vi "保存下载配置.vi"(10 "输入数组":string[][](array[string])) -> ()   [LabVIEW 2016]
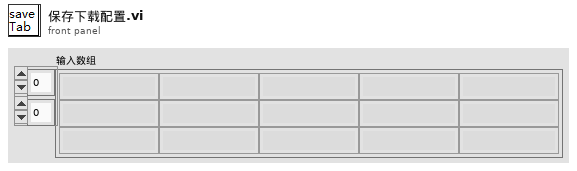
[diagram p1: front panel]
types:
  T1 = enum16{"open", "replace", "create", "open or create", "replace or create", "replace or create with confirmation"}
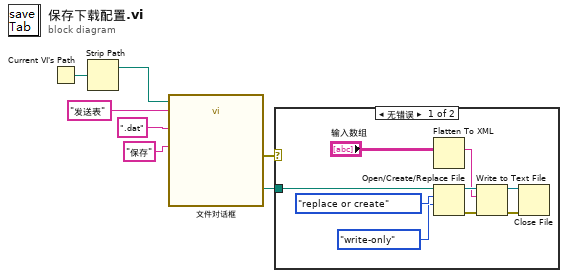
[diagram p0: block diagram]
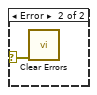
[diagram p2: hidden frame]
diagram:
  n1 = Current VI's Path() -> (path=w7:path)
  n2 = Strip Path(path=w7) -> (stripped path=w1:path)  [unwired: 1 out]
  n3 = call "文件对话框"("start path"=w1, "button label"="保存", "default name"="发送表" ("名称或相对路径"), "pattern (all files)"=".dat") -> ("selected path"=w3:path, "error out"=w2:errorcluster)  [unwired: 8 in, 2 out]
  n4 = case shown="无错误" w2 {
    selector: w2 -> [_ w17]
    tunnel: w3 -> [w16 _]
    frame No Error {
      n5 = Flatten To XML(anything="输入数组") -> (xml string=w9:string)
      n6 = Open/Create/Replace File(file path (use dialog)=w16, operation (0:open)=T1."replace or create" ("操作(0:open)"), access (0:read/write)=enum16{"read/write", "read-only", "write-only"}."write-only" ("权限(0:read/write)")) -> (refnum out=w13:refnum<file>, error out=w12:errorcluster)  [unwired: 3 in, 1 out]
      n7 = Write to Text File(file (use dialog)=w13, text=w9, error in=w12) -> (refnum out=w11:refnum<file>, error out=w10:errorcluster)  [unwired: 1 in, 1 out]
      n8 = Close File(refnum=w11, error in=w10) -> ()  [unwired: 2 out]
    }
    frame Error {
      n9 = call <vilib>:"Clear Errors.vi"("error in (no error)"=w17) -> ()  [unwired: 5 in, 2 out]
    }
  }
